vi "Append Segments.vi"(8 "error in":errorcluster, 10 "Segments":u8[](array[numeric]) format="%.0x", 11 "Segmented Upload Transfer in":refnum<class "Segmented Upload Transfer.lvclass">) -> (0 "error out":errorcluster, 3 "Segmented Upload Transfer out":refnum<class "Segmented Upload Transfer.lvclass">)   [LabVIEW 2020, in "SDO Manager.lvlib" / "Segmented Upload Transfer.lvclass"]
uses:
  Segmented Upload Transfer.lvclass
  Segmented Upload Transfer.lvclass/Segmented Upload Transfer.ctl
  D:/git/CANopen-LabVIEW/source/SDO Manager/SDO Transfer/SDO Transfer.lvclass
  D:/git/CANopen-LabVIEW/source/SDO Manager/Segmented Upload Transfer/Segmented Upload Transfer.lvclass
  SDO Transfer/SDO Transfer.lvclass
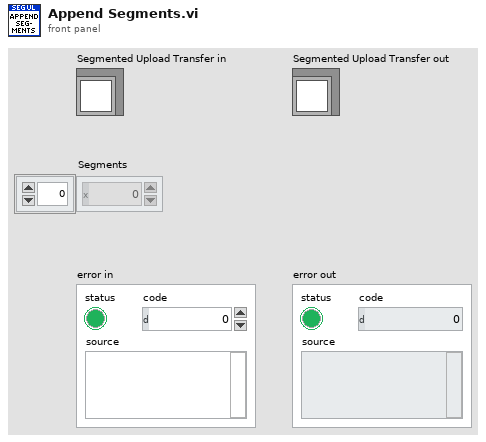
[diagram p1: front panel]
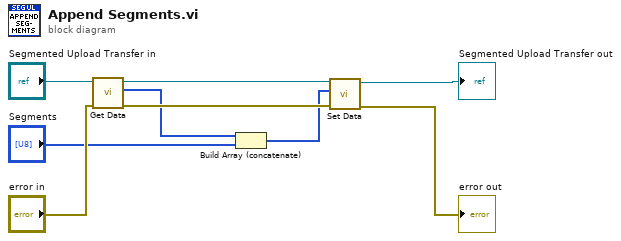
[diagram p0: block diagram]
diagram:
  n1 = call "Get Data.vi"("error in"="error in", "SDO Transfer in"="Segmented Upload Transfer in") -> ("error out"=w7:errorcluster, "Data"=w4:u8[], "SDO Transfer out"=w5:refnum<class "Segmented Upload Transfer.lvclass">)  [unwired: 7 in]
  n2 = Build Array (concatenate)(w4, "Segments") -> (w1:u8[])
  n3 = call "Set Data.vi"("error in"=w7, "Data"=w1, "SDO Transfer in"=w5) -> ("error out"=→"error out":errorcluster, "SDO Transfer out"=→"Segmented Upload Transfer out":refnum<class "Segmented Upload Transfer.lvclass">)  [unwired: 7 in]
